vi "WPI_CameraGet Image To PC Port.vi"() -> (0 "port":u16)   [LabVIEW 2017]
doc: "This software is licensed. Open the labview\\readme\\WPI Robotics Library Open Source License.txt file for more information."
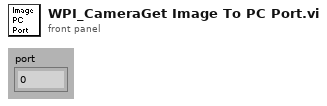
[diagram p1: front panel]
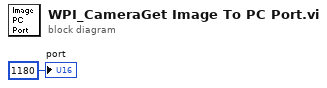
[diagram p0: block diagram]
diagram:
  "port" <- u16 1180 ("port")
